vi "PDashPathHistory--constant.vi"() -> (3 "PDashPathHistory":string)   [LabVIEW 2019, in "Panther Dashboard.lvlib"]
uses:
  Panther Dashboard.lvlib
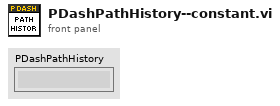
[diagram p1: front panel]
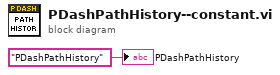
[diagram p0: block diagram]
diagram:
  "PDashPathHistory" <- "PDashPathHistory" ("key")
